vi "Read Focus ROI.vi"(8 "error in (no error)":errorcluster, 11 "Analyze Results q-Factor in":refnum<class "Analyze Results q-Factor.lvclass">) -> (0 "error out":errorcluster, 2 "ROI Descriptor":T1 {"Contours"."Type" items=["No Selection", "Point", "Line", "Rectangle", "Oval", "Polygon", "Freehand Region", "Annulus", "Unused2", "Unused3", "Broken Line", "Freehand Line", "Rotated Rectangle"]}, 3 "Analyze Results q-Factor out":refnum<class "Analyze Results q-Factor.lvclass">)   [LabVIEW 2014, in "Analyze Results q-Factor.lvclass"]
uses:
  Analyze Results q-Factor.lvclass
  Analyze Results q-Factor.lvclass/Analyze Results q-Factor.ctl
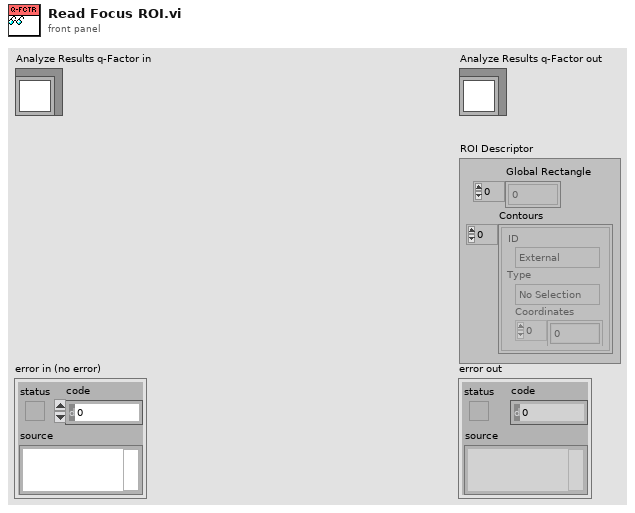
[diagram p1: front panel]
types:
  T1 = typedef "ROI Descriptor" = cluster{"Global Rectangle":i32[], "Contours":cluster{"ID":enum32{"External", "Internal"}, "Type":u32, "Coordinates":i32[]}[]}
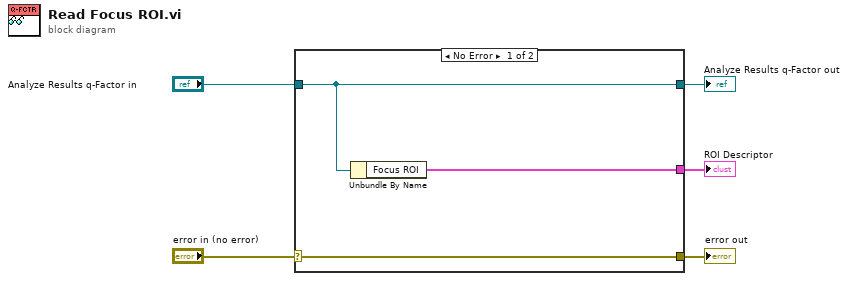
[diagram p0: block diagram]
diagram:
  n1 = case shown="No Error" "error in (no error)" {
    selector: "error in (no error)" -> [w8 w9]
    tunnel: [w8 w9] -> w4
    tunnel: [w7 w10] -> w2
    tunnel: "Analyze Results q-Factor in" -> [w7 w10]
    tunnel: [w6 _] -> w1
    frame No Error {
      n2 = Unbundle By Name(w7) -> ("Focus ROI"=w6:T1)
    }
    frame Error {
    }
  }
  "error out" <- w4
  "Analyze Results q-Factor out" <- w2
  "ROI Descriptor" <- w1
